vi "Load Classes From Relative Paths File.vi"(0 "Class Loader in":refnum<class "Class Loader.lvclass">, 5 "Caller Enqueuer":refnum<class "Message Enqueuer.lvclass">, 7 "Class Relative Paths Path":path, 9 "Reference Class Path":path, 11 "error in":errorcluster) -> (4 "Class Loader out":refnum<class "Class Loader.lvclass">, 6 "Classes Map":T1, 8 "Class Names":string[](array[string]), 10 "Class Array":refnum<class>[](array[class]), 15 "error out":errorcluster)   [LabVIEW 2023, in "Class Loader.lvlib" / "Class Loader.lvclass"]
uses:
  Class Loader.lvclass
  <vilib>/ActorFramework/Message Enqueuer/Message Enqueuer.lvclass
  Class Loader Messages/Class Loading Progress Msg/Class Loading Progress Msg.lvclass/Class Loading Progress Msg.ctl
  <vilib>/ActorFramework/Message Enqueuer/Message Enqueuer.lvclass/Message Enqueuer.ctl
  Class Loader Messages/Class Loading Progress Msg/Class Loading Progress Msg.lvclass
  C:/Program Files/National Instruments/LabVIEW 2025/vi.lib/ActorFramework/Message/Message.lvclass
  Class Loader.lvclass/Class Loader.ctl
  Class Details.ctl
  ced2505d-d48f-485f-802f-01d2a2dbf5ba.vi
  Classes Map.ctl
  <vilib>/Utility/miscctls.llb/LVMapReplaceAction.ctl
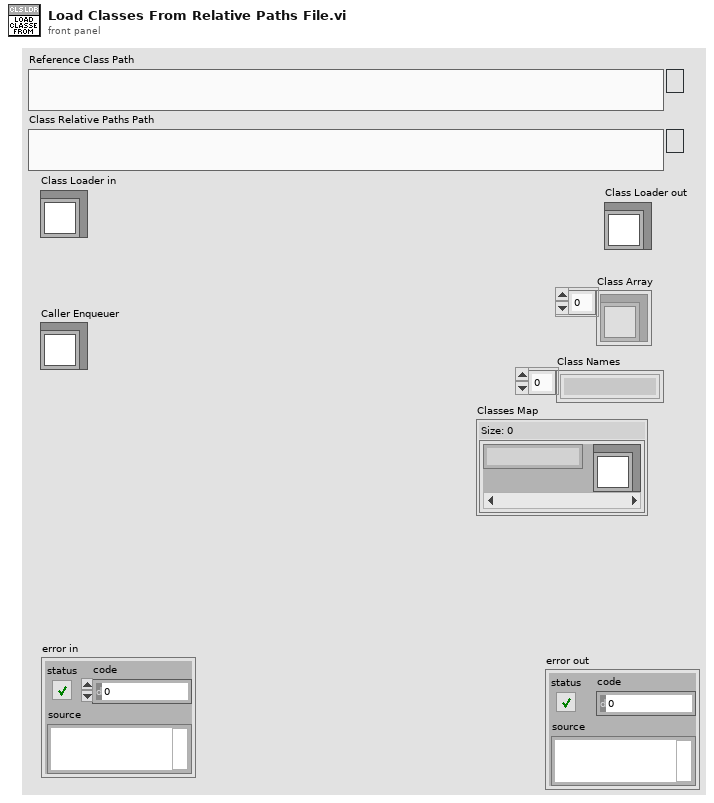
[diagram p1: front panel]
types:
  T1 = typedef "Class Loader.lvlib/Class Loader.lvclass/Classes Map.ctl" = map{string, refnum<class>}
  T2 = enum16{"open", "replace", "create", "open or create", "replace or create", "replace or create with confirmation"}
  T3 = typedef "Class Loader.lvlib/Class Loader.lvclass/Classes Cache Map.ctl" = map{path, refnum<class>}
  T4 = typedef "Class Loader.lvlib/Class Loader.lvclass/Class Details.ctl" = cluster{"Class Name":string, "Class":refnum<class>}
  T5 = typedef "LVMapReplaceAction.ctl" = enum32{"Modify Entry only if found", "Add or Modify Entry", "Delete Entry"}
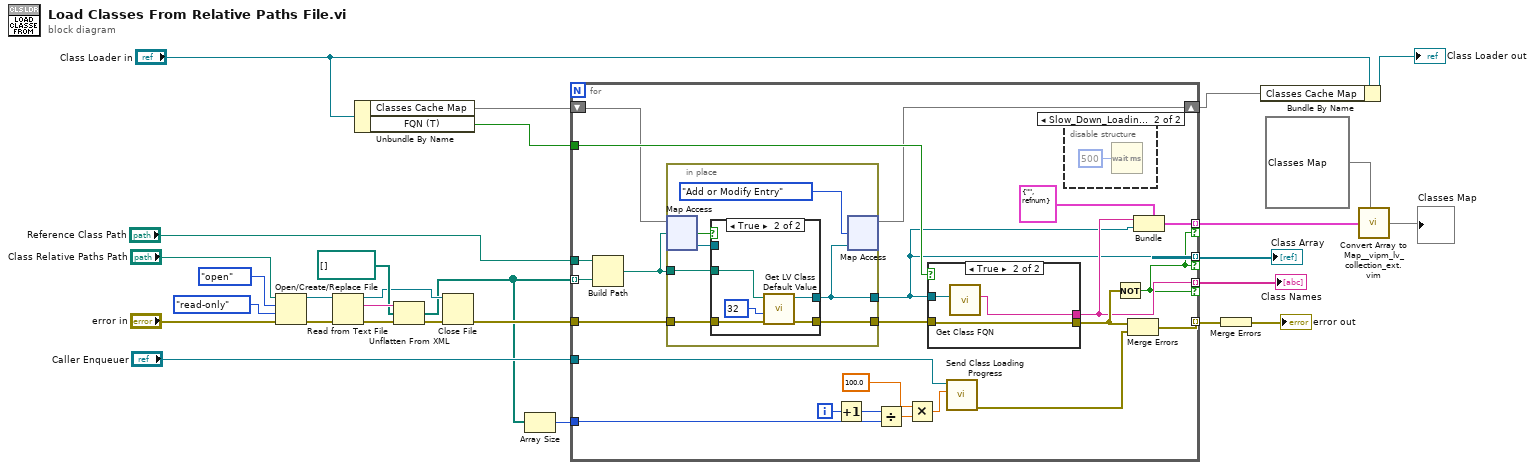
[diagram p0: block diagram]
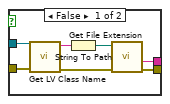
[diagram p3: hidden frame]
diagram:
  n1 = Open/Create/Replace File(file path (use dialog)="Class Relative Paths Path", error in="error in", operation (0:open)=T2."open", access (0:read/write)=enum16{"read/write", "read-only", "write-only"}."read-only") -> (refnum out=w24:refnum<file>, error out=w25:errorcluster)  [unwired: 2 in, 1 out]
  n2 = Read from Text File(file (use dialog)=w24, error in=w25) -> (refnum out=w19:refnum<file>, text=w23:string, error out=w21:errorcluster)  [unwired: 2 in, 1 out]
  n3 = Unbundle By Name("Class Loader in") -> ("Classes Cache Map"=w5:T3, "FQN (T)"=w1:bool)
  n4 = Unflatten From XML(xml string=w23, type=path[] [], error in (no error)=w21) -> (value=w10:path[], error out=w20:errorcluster)
  n5 = Close File(refnum=w19, error in=w20) -> (error out=w16:errorcluster)  [unwired: 1 out]
  n6 = Array Size(array=w10) -> (size(s)=w9:i32)
  n7 = for {
    tunnel: w10 -> [w50] mode=indexing
    tunnel: [w32] -> w18 mode=indexing if=w45
    tunnel: "Reference Class Path" -> [w51]
    tunnel: w16 -> [w31]
    tunnel: [w37] -> w15 mode=indexing
    tunnel: [w47] -> w13 mode=indexing if=w45
    tunnel: [w46] -> w7 mode=indexing if=w45
    tunnel: "Caller Enqueuer" -> [w38]
    tunnel: w9 -> [w42]
    tunnel: w1 -> [w35]
    shift-right: [w29] -> w2
    shift-left: w5 -> [w34]
    i -> [w44]
    n8 = Build Path(base path=w51, name or relative path=w50) -> (appended path=w33:path)
    n9 = in-place {
      in-place-border: w33 -> [w57]
      in-place-border: [w52] -> w32
      in-place-border: w31 -> [w56]
      in-place-border: [w55] -> w30
      n10 = in-place-map #1(w34, w33) -> (w53:refnum<class>, w54:bool)  [unwired: 1 in]
      n11 = case shown="True" w54 {
        tunnel: w57 -> [_ w64]
        tunnel: [w60 w63] -> w52
        tunnel: w56 -> [w59 w62]
        tunnel: [w59 w61] -> w55
        tunnel: w53 -> [w60 _]
        frame False {
        }
        frame True {
          n12 = call <vilib>:"Get LV Class Default Value.vi"("error in (no error)"=w62, "options"=u32 32, "class path"=w64) -> ("error out"=w61:errorcluster, "object"=w63:refnum<class>)  [unwired: 7 in]
        }
      }
      n13 = in-place-map #1(w52, LVMapReplaceAction."Add or Modify Entry" ("action")) -> (w29:T3)  [unwired: 2 out]
    }
    n14 = Increment(x=w44) -> (x+1=w43:i32)
    n15 = Divide(x=w43, y=w42) -> (x/y=w41:dbl)
    n16 = Multiply(x=100.0, y=w41) -> (x*y=w39:dbl)
    n17 = case shown="True" w35 {
      tunnel: w30 -> [w69 w74]
      tunnel: [w68 w74] -> w49
      tunnel: [w67 w73] -> w47
      tunnel: w32 -> [w66 w75]
      frame False {
        n18 = call <vilib>:"Get LV Class Name.vi"("error in (no error)"=w69, "object"=w66) -> ("error out"=w72:errorcluster, "class name"=w70:string)  [unwired: 8 in]
        n19 = String To Path(string=w70) -> (path=w71:path)
        n20 = call <vilib>:"Get File Extension.vi"("error in (no error)"=w72, "file"=w71) -> ("error out"=w68:errorcluster, "filename without extension"=w67:string)  [unwired: 5 in, 3 out]
      }
      frame True {
        n21 = call "Get Class FQN.vi"("LabVIEW Object"=w75) -> ("QualifiedName"=w73:string)  [unwired: 10 in]
      }
    }
    n22 = call "Send Class Loading Progress.vi"("Progress (%)"=w39, "Message Enqueuer in"=w38) -> ("error out"=w36:errorcluster)  [unwired: 8 in, 1 out]
    n23 = disable-structure shown="Slow_Down_Loading==True" {
      frame condition #0 (active) {
      }
      frame condition #1 {
        n24 = Wait (ms)(milliseconds to wait=u32 500) -> ()  [unwired: 1 out]
      }
    }
    n25 = Not(x=w49) -> (.not. x?=w45:bool)
    n26 = Merge Errors(w49, w36) -> (w37:errorcluster)
    n27 = Bundle(cluster=T4 {"Class Name"="", "Class"=refnum} ("Class Details"), "Class Name"=w47, "Class"=w32) -> (w46:T4)
  }
  "Class Array" <- w18
  "Class Names" <- w13
  n28 = Merge Errors(w15) -> (→"error out":errorcluster)
  n29 = Bundle By Name(cluster="Class Loader in", "Classes Cache Map"=w2) -> (→"Class Loader out":refnum<class "Class Loader.lvclass">)
  n30 = call "Convert Array to Map__vipm_lv_collection_ext.vim"("map type (optional)"=T1 {} ("Classes Map"), "array"=w7) -> ("map"=→"Classes Map":T1)  [unwired: 5 in]
